vi "Save Data Sets.vi"(8 "error in (no error)":errorcluster, 10 "Information":T1, 11 "Saving Path":path) -> (0 "error out":errorcluster)   [LabVIEW 2020]
uses:
  <vilib>/Utility/config.llb/Write Key (Double).vi
  <vilib>/Utility/config.llb/Write Key (Boolean).vi
  <vilib>/Utility/config.llb/Write Key (String).vi
  <vilib>/Utility/config.llb/NI_LVConfig.lvlib
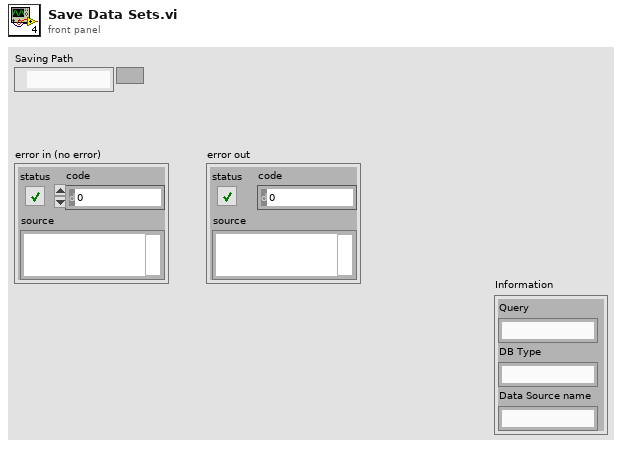
[diagram p1: front panel]
types:
  T1 = cluster{"Query":string, "DB Type":string, "Data Source name":string}
  T2 = typedef "NI_LVConfig.lvlib/Config Data RefNum.ctl" = refnum<k1>
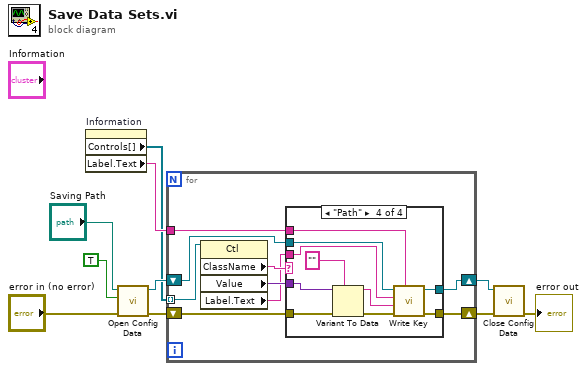
[diagram p0: block diagram]
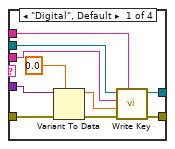
[diagram p2: hidden frame]
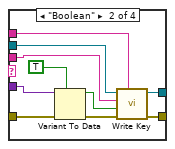
[diagram p3: hidden frame]
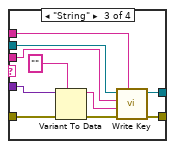
[diagram p4: hidden frame]
diagram:
  n1 = property on="Information" class="Clust (strict)"() -> ("Controls[]"=w1:refnum<vi>[], "Label.Text"=w2:string)  [unwired: 2 in, 2 out]
  n2 = call <vilib>:"Open Config Data.vi"("error in (no error)"="error in (no error)", "create file if necessary (T)"=TRUE, "configuration file path"="Saving Path") -> ("error out"=w5:errorcluster, "refnum"=w4:T2)  [unwired: 6 in, 1 out]
  n3 = for {
    shift-right: [w14] -> w7
    shift-left: w5 -> [w16]
    shift-right: [w13] -> w6
    shift-left: w4 -> [w15]
    tunnel: w2 -> [w17]
    tunnel: w1 -> [w19] mode=indexing
    n4 = property class="Ctl"(reference=w19) -> ("ClassName"=w18:string, "Value"=w12:variant, "Label.Text"=w11:string)  [unwired: 1 in, 2 out]
    n5 = case shown="\"Path\"" w18 {
      tunnel: w17 -> [w23 w39 w49 w59]
      tunnel: w16 -> [w26 w34 w44 w54]
      tunnel: w15 -> [w22 w38 w48 w58]
      tunnel: [w25 w37 w47 w57] -> w14
      tunnel: [w24 w36 w46 w56] -> w13
      tunnel: w12 -> [w27 w35 w45 w55]
      tunnel: w11 -> [w21 w30 w41 w51]
      frame "Digital", Default {
        n6 = Variant To Data(error in=w26, type=0.0, Variant=w27) -> (data=w28:dbl, error out=w29:errorcluster)
        n7 = call-poly <vilib>:"Write Key.vi"("section"=w23, "error in (no error)"=w29, "value"=w28, "key"=w21, "refnum"=w22) -> ("error out"=w25:errorcluster, "refnum out"=w24:T2)  [unwired: 4 in, 1 out]
      }
      frame "Boolean" {
        n8 = Variant To Data(error in=w34, type=TRUE, Variant=w35) -> (data=w31:bool, error out=w33:errorcluster)
        n9 = call-poly <vilib>:"Write Key.vi"("section"=w39, "error in (no error)"=w33, "value"=w31, "key"=w30, "refnum"=w38) -> ("error out"=w37:errorcluster, "refnum out"=w36:T2)  [unwired: 4 in, 1 out]
      }
      frame "String" {
        n10 = Variant To Data(error in=w44, type="", Variant=w45) -> (data=w42:string, error out=w43:errorcluster)
        n11 = call-poly <vilib>:"Write Key.vi"("section"=w49, "error in (no error)"=w43, "value"=w42, "key"=w41, "refnum"=w48) -> ("error out"=w47:errorcluster, "refnum out"=w46:T2)  [unwired: 4 in, 1 out]
      }
      frame "Path" {
        n12 = Variant To Data(error in=w54, type="", Variant=w55) -> (data=w52:string, error out=w53:errorcluster)
        n13 = call-poly <vilib>:"Write Key.vi"("section"=w59, "error in (no error)"=w53, "value"=w52, "key"=w51, "refnum"=w58) -> ("error out"=w57:errorcluster, "refnum out"=w56:T2)  [unwired: 4 in, 1 out]
      }
    }
  }
  n14 = call <vilib>:"Close Config Data.vi"("error in (no error)"=w7, "refnum"=w6) -> ("error out"=→"error out":errorcluster)  [unwired: 8 in, 1 out]
